vi "AVeryComplexVI.vi"(8 "Error In":errorcluster) -> (0 "Error Out":errorcluster)   [LabVIEW 2019]
panel:
  out "Boolean":bool
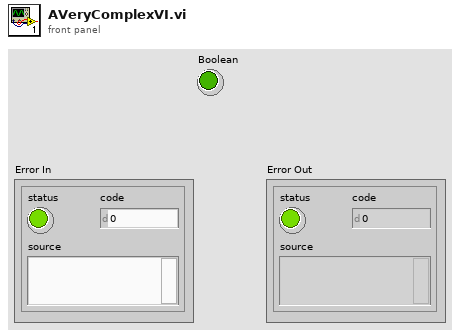
[diagram p1: front panel]
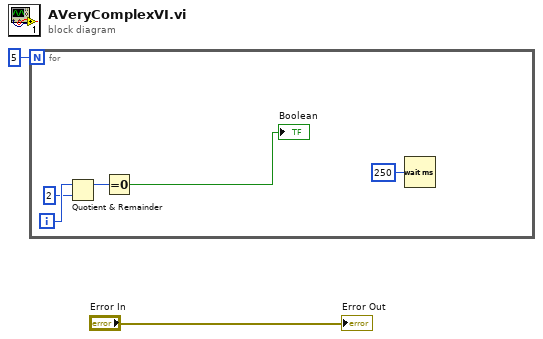
[diagram p0: block diagram]
diagram:
  n1 = for {
    N: 5 -> [_]
    i -> [w7]
    n2 = Quotient & Remainder(x=w7, y=2) -> (x-y*floor(x/y)=w6:i32)  [unwired: 1 out]
    n3 = Equal To 0?(x=w6) -> (x = 0?=→"Boolean":bool)
    n4 = Wait (ms)(milliseconds to wait=u32 250) -> ()  [unwired: 1 out]
  }
  "Error Out" <- "Error In"
